vi "ReadArray.vi"(8 "error in (no error)":errorcluster, 9 "Keithley Config":T1={"Source Compliance (A)"=0.1, "Min Voltage (V)"=0.0, "Max Voltage (V)"=5.0, "Source Mode"=0, "Number of Points"=50} {"Number of Points" min=2 step=1; "Source Mode" items=["Voltage", "Current"]; "Min Voltage (V)" min=0.1}, 10 "t0 2":dbl, 11 "VISA resource name":refnum<visa-resource-name>) -> (0 "error out":errorcluster, 1 "Resistance (ohm)":dbl[](array[numeric]), 2 "appended array":sgl[][](array[numeric]), 3 "VISA resource name out":refnum<visa-resource-name>)   [LabVIEW 2019, in "SMU.lvclass"]
uses:
  SMU.lvclass
  typeDefs/keithleySettings.ctl
panel:
  out "x-y":dbl
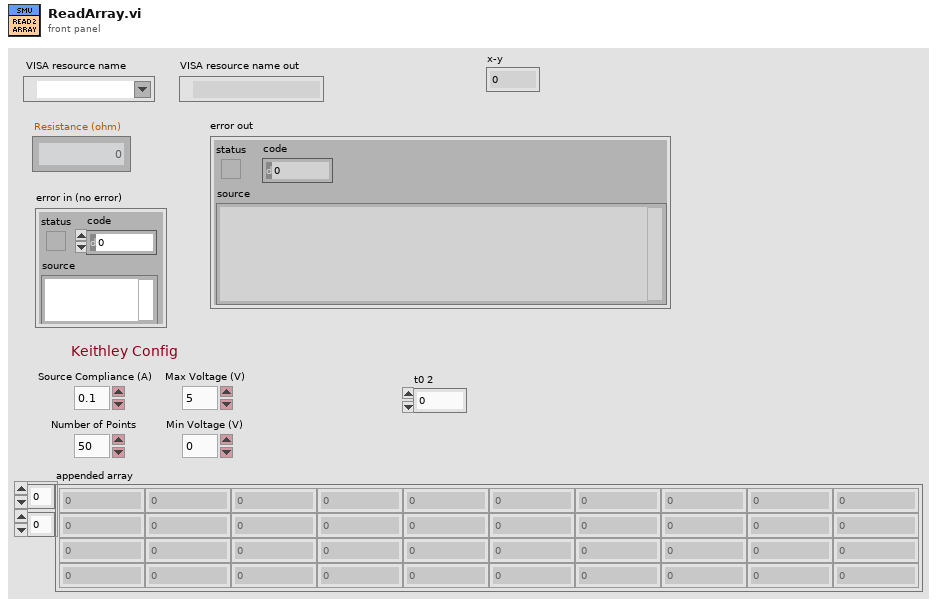
[diagram p1: front panel]
types:
  T1 = typedef "keithleySettings.ctl" = cluster{"Source Compliance (A)":dbl, "Min Voltage (V)":dbl, "Max Voltage (V)":dbl, "Source Mode":u16, "Number of Points":u32}
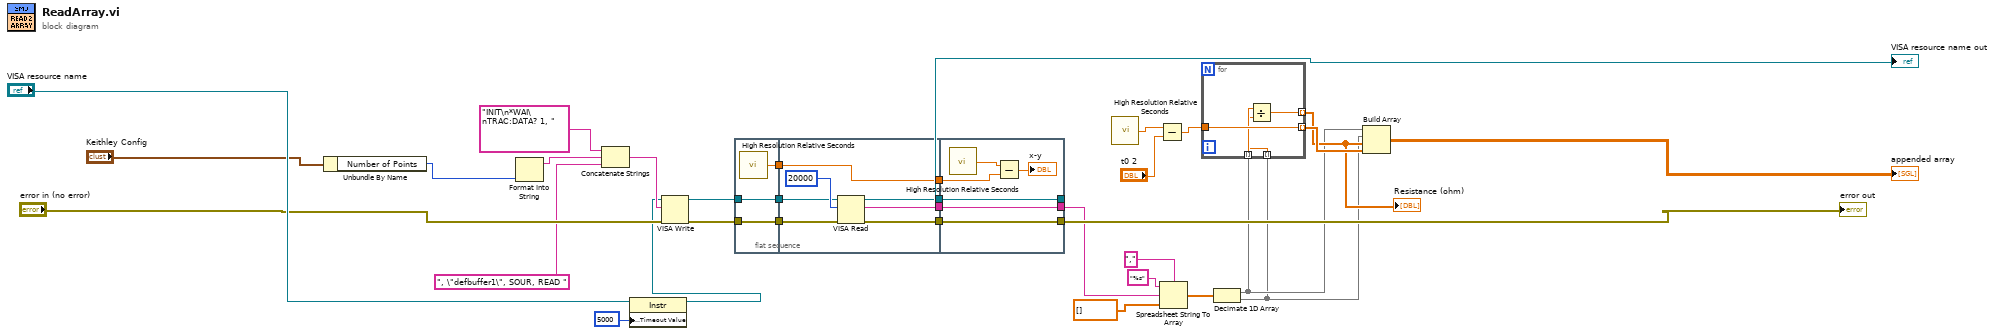
[diagram p0: block diagram]
diagram:
  n1 = Unbundle By Name("Keithley Config") -> ("Number of Points"=w14:u32)
  n2 = Format Into String(w14) -> (resulting string=w12:string)  [unwired: 3 in, 1 out]
  n3 = Concatenate Strings("INIT\n*WAI\nTRAC:DATA? 1, ", w12, ", \"defbuffer1\", SOUR, READ " ("string")) -> (w10:string)
  n4 = property class="Instr"(reference="VISA resource name", "General Settings:Timeout Value"=u32 5000) -> (reference out=w9:refnum<visa-resource-name>)  [unwired: 1 in, 1 out]
  n5 = VISA Write(VISA resource name=w9, write buffer=w10, error in (no error)="error in (no error)") -> (VISA resource name out=w22:refnum<visa-resource-name>, error out=w23:errorcluster)  [unwired: 1 out]
  n6 = flat-sequence {
    tunnel: w22 -> [w36]
    tunnel: w23 -> [w37]
    tunnel: [w37] -> w4
    tunnel: [w36] -> w3
    tunnel: [w35] -> w2
    tunnel: [w44] -> w7
    tunnel: [w43] -> w6
    tunnel: [w39] -> w5
    tunnel: w4 -> [w41]
    tunnel: w3 -> [w40]
    tunnel: w2 -> [w38]
    tunnel: [w38] -> w1
    tunnel: [w48] -> w17
    tunnel: [w49] -> w30
    tunnel: [w50] -> w31
    tunnel: w7 -> [w50]
    tunnel: w6 -> [w49]
    tunnel: w5 -> [w48]
    tunnel: w1 -> [w46]
    frame #0 {
      n7 = call <vilib>:"High Resolution Relative Seconds.vi"() -> ("relative seconds"=w35:dbl)
    }
    frame #1 {
      n8 = VISA Read(VISA resource name=w40, byte count=u32 20000, error in (no error)=w41) -> (VISA resource name out=w43:refnum<visa-resource-name>, read buffer=w39:string, error out=w44:errorcluster)  [unwired: 1 out]
    }
    frame #2 {
      n9 = call <vilib>:"High Resolution Relative Seconds.vi"() -> ("relative seconds"=w47:dbl)
      n10 = Subtract(x=w47, y=w46) -> (x-y=→"x-y":dbl)
    }
  }
  n11 = call <vilib>:"High Resolution Relative Seconds.vi"() -> ("relative seconds"=w25:dbl)
  n12 = Subtract(x=w25, y="t0 2") -> (x-y=w28:dbl)
  n13 = Spreadsheet String To Array(delimiter (Tab)=",", format string="%s", spreadsheet string=w17, array type (2D Dbl)=dbl[] []) -> (array=w18:dbl[])
  n14 = Decimate 1D Array(w18) -> (w16:dbl[], w15:dbl[])
  n15 = for {
    tunnel: [w54] -> w26 mode=indexing
    tunnel: w28 -> [w53]
    tunnel: [w53] -> w27 mode=indexing
    tunnel: w16 -> [w52] mode=indexing
    tunnel: w15 -> [w51] mode=indexing
    n16 = Divide(x=w52, y=w51) -> (x/y=w54:dbl)
  }
  "Resistance (ohm)" <- w26
  n17 = Build Array(w16, w15, w26, w27) -> (→"appended array":dbl[][])
  "error out" <- w31
  "VISA resource name out" <- w30
